vi "MeasureJoule.vi"(5 "Junction Name":string, 6 "UiDefinition":T1, 7 ".NET Refnum":refnum<k24>, 8 "new file path (Not A Path if cancelled)":path, 10 "appended path":path, 11 ".NET Refnum in":refnum<k24>) -> (0 "error out":errorcluster, 3 "Cluster":cluster{dbl[], dbl[]})   [LabVIEW 2020]
uses:
  UIReferences.ctl
  C:/Users/User/Desktop/Automation/CurrentVersion/LabviewDXFViewer/bin/Release/LabviewDXFViewer.exe
  LabviewDXFViewer/bin/Release/LabviewDXFViewer.exe
  <vilib>/Utility/file.llb/Write Delimited Spreadsheet (string).vi
  <vilib>/Utility/file.llb/Write Delimited Spreadsheet (DBL).vi
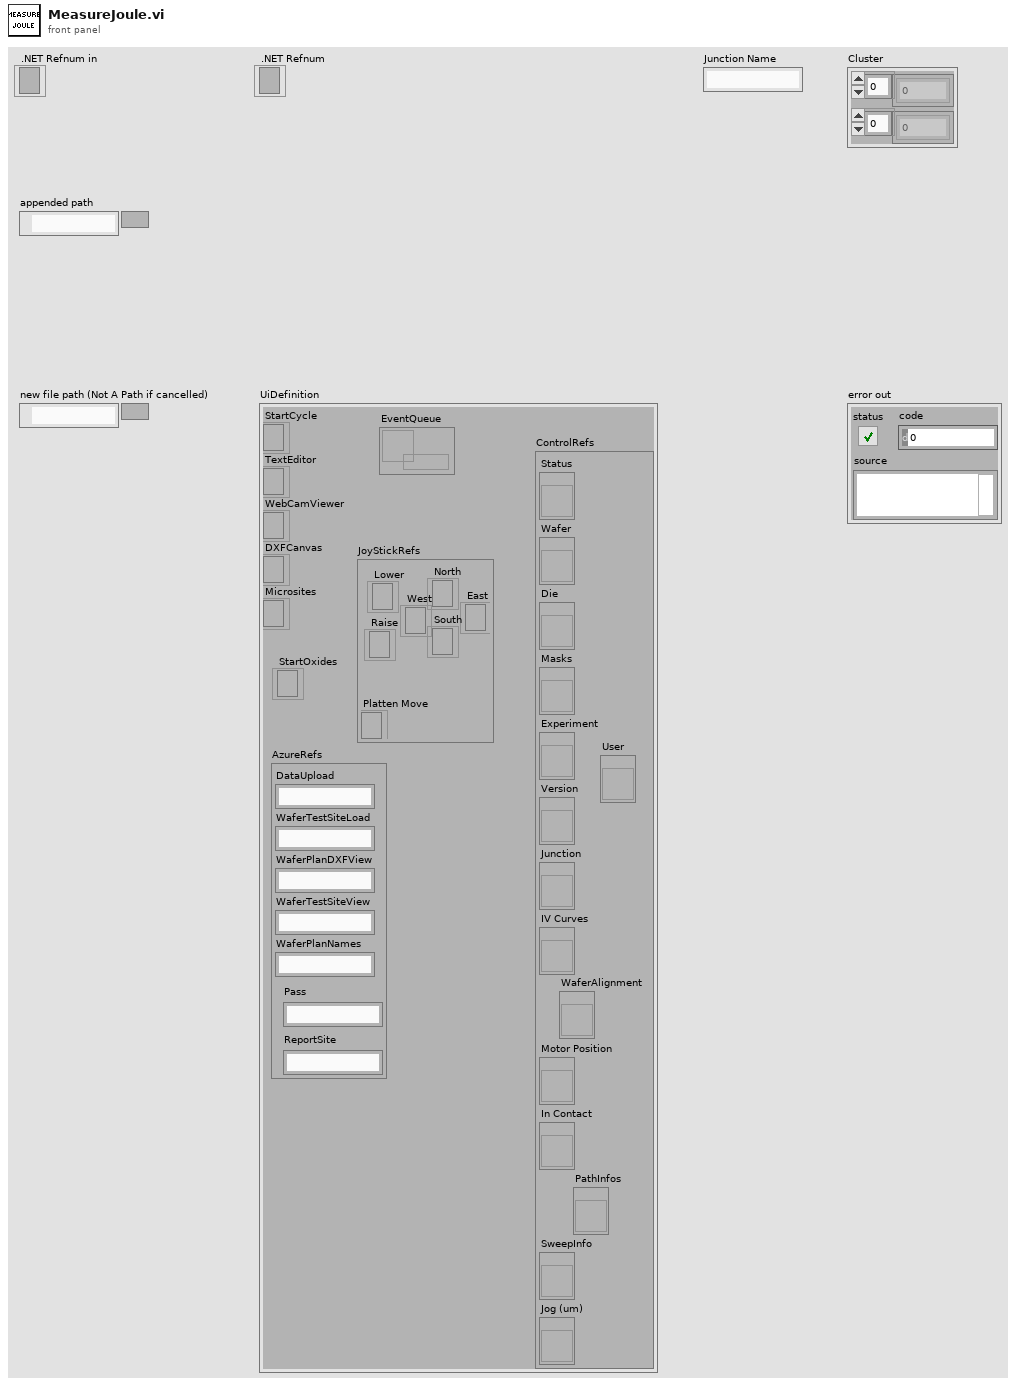
[diagram p1: front panel]
types:
  T1 = typedef "UIReferences.ctl" = cluster{"StartCycle":refnum<k24>, "TextEditor":refnum<k24>, "WebCamViewer":refnum<k24>, "DXFCanvas":refnum<k24>, "Microsites":refnum<k24>, "JoyStickRefs":cluster{"North":refnum<k24>, "Lower":refnum<k24>, "Raise":refnum<k24>, "Platten Move":refnum<k24>, "West":refnum<k24>, "East":refnum<k24>, "South":refnum<k24>}, "AzureRefs":cluster{"DataUpload":string, "WaferTestSiteLoad":string, "WaferPlanDXFView":string, "WaferTestSiteView":string, "WaferPlanNames":string, "Pass":string, "ReportSite":string}, "ControlRefs":cluster{"Status":refnum<vi>, "Wafer":refnum<vi>, "Die":refnum<vi>, "Masks":refnum<vi>, "Experiment":refnum<vi>, "Version":refnum<vi>, "Junction":refnum<vi>, "IV Curves":refnum<vi>, "Motor Position":refnum<vi>, "In Contact":refnum<vi>, "SweepInfo":refnum<vi>, "Jog (um)":refnum<vi>, "PathInfos":refnum<vi>, "User":refnum<vi>, "WaferAlignment":refnum<vi>}, "EventQueue":refnum<queue>, "StartOxides":refnum<k24>}
  T2 = typedef "CapacitanceInfos.ctl" = cluster{"Conductance":dbl, "CapacitanceIV":dbl, "Intercept":dbl, "CapacitanceSW":dbl, "Sum":dbl, "CapacitanceInfos":T3[], "CapacitancePhase":dbl, "dC/dV":dbl}
  T3 = typedef "CapacitanceRecord.ctl" = cluster{"Freq":dbl, "Vpp":dbl, "PhaseS":dbl, "Irms":dbl, "PhaseC":dbl, "Theta":dbl, "VDrive":dbl, "Capacitance":dbl, "Other":dbl}
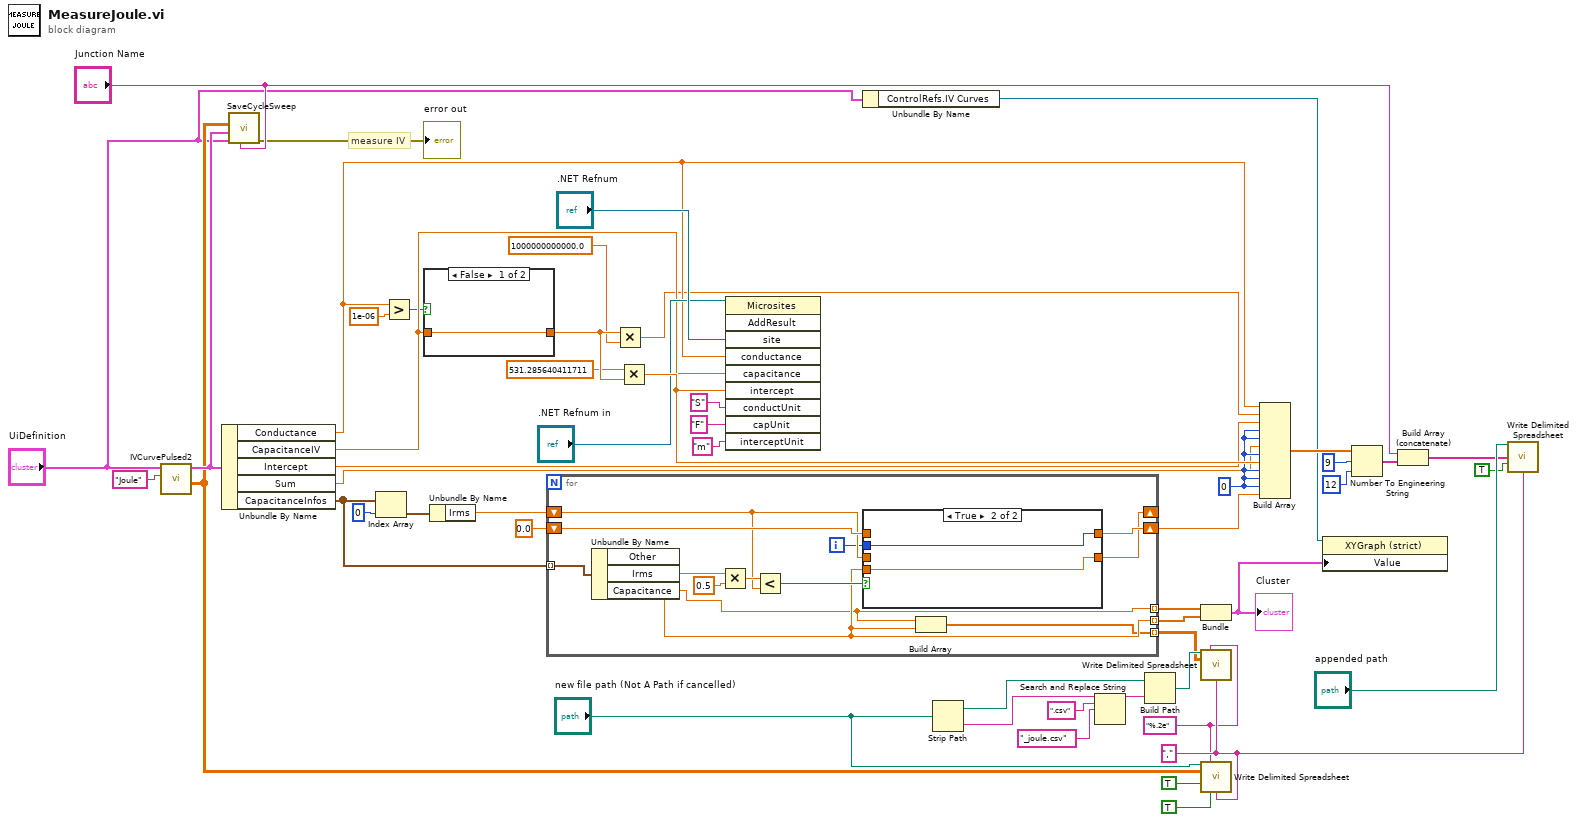
[diagram p0: block diagram]
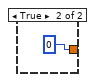
[diagram p3: hidden frame]
diagram:
  w5 = "," ("delimiter (\\t)")
  w49 = 0
  w4 = "%.2e" ("format (%.3f)")
  # "measure IV"
  n1 = call "IVCurvePulsed2.vi"("Program"="Joule", "UiDefinition"="UiDefinition") -> ("appended array"=w21:dbl[][], "InfoCluster"=w34:T2)  [unwired: 8 in]
  n2 = Unbundle By Name(w34) -> ("Conductance"=w36:dbl, "CapacitanceIV"=w35:dbl, "Intercept"=w24:dbl, "Sum"=w25:dbl, "CapacitanceInfos"=w39:T3[])
  n3 = call "SaveCycleSweep.vi"("JunctionName"="Junction Name", "UiDefinition 2"="UiDefinition", "InfoCluster"=w34, "appended array"=w21) -> ("error out"=→"error out":errorcluster)  [unwired: 7 in]
  n4 = Index Array(array=w39, index=0) -> (element=w41:T3)
  n5 = Greater?(x=w36, y=1e-06) -> (0:w28:bool)
  n6 = case shown="False" w28 {
    tunnel: [w53 0] -> w51
    tunnel: w35 -> [w53 _]
    frame False {
    }
    frame True {
    }
  }
  n7 = Unbundle By Name(w41) -> ("Irms"=w42:dbl)
  n8 = for {
    tunnel: w39 -> [w66] mode=indexing
    tunnel: [w55] -> w37 mode=indexing
    tunnel: [w57] -> w38 mode=indexing
    shift-right: [w59] -> _
    shift-left: w42 -> [w60]
    shift-right: [w64] -> w48
    shift-left: 0.0 ("Vpp") -> [w63]
    tunnel: [w56] -> w6 mode=indexing
    i -> [w58]
    n9 = Unbundle By Name(w66) -> ("Irms"=w57:dbl, "Capacitance"=w55:dbl)  [unwired: 1 out]
    n10 = Multiply(x=w57, y=0.5) -> (x*y=w62:dbl)
    n11 = Less?(x=w62, y=w60) -> (x < y?=w65:bool)
    n12 = case shown="True" w65 {
      tunnel: w58 -> [_ w70]
      tunnel: [w68 w70] -> w64
      tunnel: w63 -> [w68 _]
      tunnel: [w67 w69] -> w59
      tunnel: w60 -> [w67 _]
      tunnel: w57 -> [_ w69]
      frame False {
      }
      frame True {
      }
    }
    n13 = Build Array(w55, w57) -> (w56:dbl[])
  }
  n14 = Multiply(x=w51, y=1000000000000.0) -> (x*y=w26:dbl)
  n15 = Multiply(x=531.285640411711, y=w51) -> (x*y=w52:dbl)
  n16 = invoke class="Microsites" method="AddResult"(reference=".NET Refnum in", "site"=".NET Refnum", "conductance"=w36, "capacitance"=w35, "intercept"=w52, "conductUnit"="S", "capUnit"="F", "interceptUnit"="m") -> ()  [unwired: 2 in, 10 out]
  n17 = Unbundle By Name("UiDefinition") -> ("ControlRefs.IV Curves"=w2:refnum<vi>)
  n18 = Strip Path(path="new file path (Not A Path if cancelled)") -> (stripped path=w9:path, name=w13:string)
  n19 = Search and Replace String(input string=w13, search string=".csv", replace string="_joule.csv" ("replace string (\"\")")) -> (result string=w10:string)  [unwired: 5 in, 3 out]
  n20 = Build Path(base path=w9, name or relative path=w10) -> (appended path=w7:path)
  n21 = Bundle(w37, w38) -> (w1:cluster{dbl[], dbl[]})  [unwired: 1 in]
  "Cluster" <- w1
  n22 = call-poly <vilib>:"Write Delimited Spreadsheet.vi"("file path (dialog if empty)"=w7, "format (%.3f)"=w4, "2D data"=w6, "delimiter (\\t)"=w5) -> ()  [unwired: 10 in, 2 out]
  n23 = call-poly <vilib>:"Write Delimited Spreadsheet.vi"("file path (dialog if empty)"="new file path (Not A Path if cancelled)", "format (%.3f)"=w4, "2D data"=w21, "append to file? (new file:F)"=TRUE, "transpose? (no:F)"=TRUE, "delimiter (\\t)"=w5) -> ()  [unwired: 8 in, 2 out]
  n24 = Build Array(w36, w26, w24, w49, w49, w25, w49, w52, w49, w49, w49, w48) -> (w23:dbl[])
  n25 = property class="XYGraph (strict)"(reference=w2, "Value"=w1) -> ()  [unwired: 1 in, 2 out]
  n26 = Number To Engineering String(2:i16 12 ("precision (6)"), 3:i16 9 ("width (-)"), 4:w23) -> (0:w16:string[])  [unwired: 1 in]
  n27 = Build Array (concatenate)("Junction Name", w16) -> (w18:string[])
  n28 = call-poly <vilib>:"Write Delimited Spreadsheet.vi"("file path (dialog if empty)"="appended path", "1D data"=w18, "append to file? (new file:F)"=TRUE, "delimiter (\\t)"=w5) -> ()  [unwired: 10 in, 2 out]
